vi "Read timeout by val.vi"(8 "error in (no error)":errorcluster, 11 "GET Async in":refnum<class "GET Async.lvclass">) -> (0 "error out":errorcluster, 2 "timeout (10000)":i32=10000, 3 "GET Async out":refnum<class "GET Async.lvclass">)   [LabVIEW 2019, in "HTTP Client Extensions.lvlib" / "GET Async.lvclass"]
uses:
  GET Async.lvclass
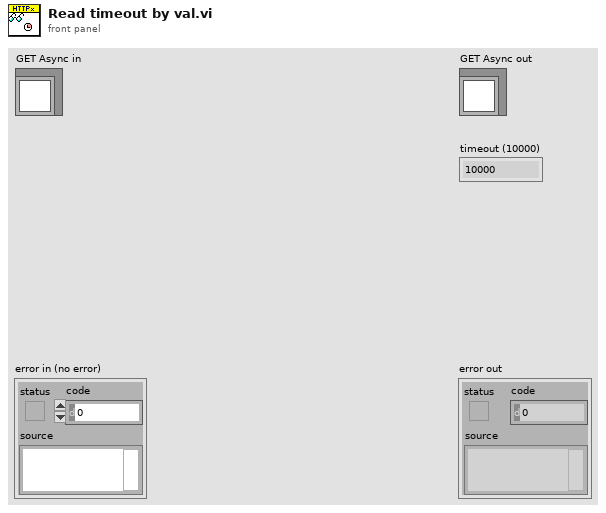
[diagram p1: front panel]
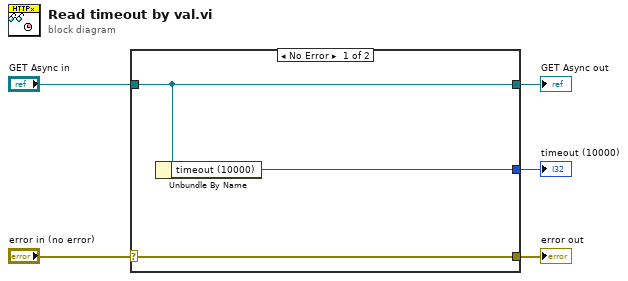
[diagram p0: block diagram]
diagram:
  n1 = case shown="No Error" "error in (no error)" {
    selector: "error in (no error)" -> [w8 w9]
    tunnel: [w8 w9] -> w4
    tunnel: [w7 w10] -> w2
    tunnel: "GET Async in" -> [w7 w10]
    tunnel: [w6 _] -> w1
    frame No Error {
      n2 = Unbundle By Name(w7) -> ("timeout (10000)"=w6:i32)
    }
    frame Error {
    }
  }
  "error out" <- w4
  "GET Async out" <- w2
  "timeout (10000)" <- w1
